vi "findMappedChannel.vi"(8 "error in (no error)":errorcluster, 10 "name of mappedTo channel":string, 11 "ChannelArray in":refnum<class "ChannelArray.lvclass">) -> (0 "error out":errorcluster, 2 "Channel":refnum<class "Channel.lvclass">, 3 "ChannelArray out":refnum<class "ChannelArray.lvclass">)   [LabVIEW 2011, in "Tools.lvlib" / "DatabaseHelpers.lvlib" / "ChannelArray.lvclass"]
uses:
  ChannelArray.lvclass
  Channel/Channel.lvclass
  ChannelArray.lvclass/ChannelArray.ctl
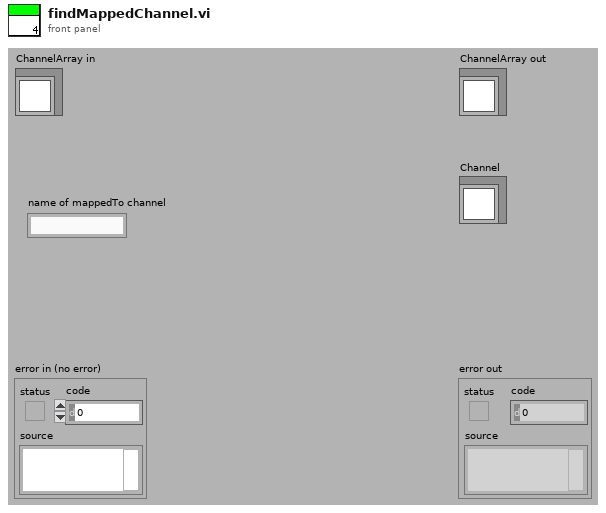
[diagram p1: front panel]
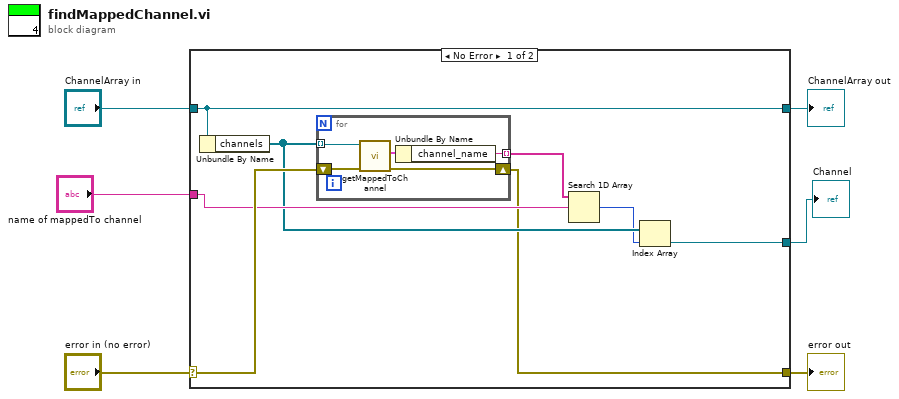
[diagram p0: block diagram]
diagram:
  n1 = case shown="No Error" "error in (no error)" {
    selector: "error in (no error)" -> [w13 w21]
    tunnel: [w7 w21] -> w5
    tunnel: [w14 w20] -> w3
    tunnel: "ChannelArray in" -> [w14 w20]
    tunnel: "name of mappedTo channel" -> [w11 _]
    tunnel: [w8 _] -> w1
    frame No Error {
      n2 = Unbundle By Name(w14) -> ("channels"=w10:refnum<class "Channel.lvclass">[])
      n3 = for {
        tunnel: w10 -> [w19] mode=indexing
        tunnel: [w17] -> w12 mode=indexing
        shift-right: [w15] -> w7
        shift-left: w13 -> [w16]
        n4 = call "getMappedToChannel.vi"("error in (no error)"=w16, "Channel.lvclass in"=w19) -> ("error out"=w15:errorcluster, "mappedTo"=w18:cluster{"type":string, "channel_name":string})  [unwired: 7 in, 1 out]
        n5 = Unbundle By Name(w18) -> ("channel_name"=w17:string)
      }
      n6 = Search 1D Array(1D array=w12, element=w11) -> (index of element=w9:i32)  [unwired: 1 in]
      n7 = Index Array(array=w10, index=w9) -> (element=w8:refnum<class "Channel.lvclass">)
    }
    frame Error {
    }
  }
  "error out" <- w5
  "ChannelArray out" <- w3
  "Channel" <- w1
